vi "Init PAS CVT.vi"(8 "error in":errorcluster, 10 "CVT Session in":T2, 11 "Cfg Ref in":T1) -> (0 "error out":errorcluster, 2 "CVT Session Out":T2, 3 "Refnum out":T1)   [LabVIEW 2014, in "Controller.lvlib" / "Controller.lvclass"]
uses:
  Controller.lvclass
  <userlib>/_Session Fwk/Typedefs/Session Handle.ctl
  <userlib>/_Session Fwk/Session - Root.lvclass
  <vilib>/Utility/config.llb/Config Data RefNum.ctl
  <vilib>/Utility/config.llb/Read Key (Boolean).vi
  <vilib>/Utility/config.llb/Read Key (I32).vi
  <vilib>/Utility/config.llb/Read Key (Double).vi
  <vilib>/Utility/config.llb/Read Key (String).vi
  <vilib>/Utility/config.llb/NI_LVConfig.lvlib
  reusable/Session APIs/CVT/CVT.lvclass
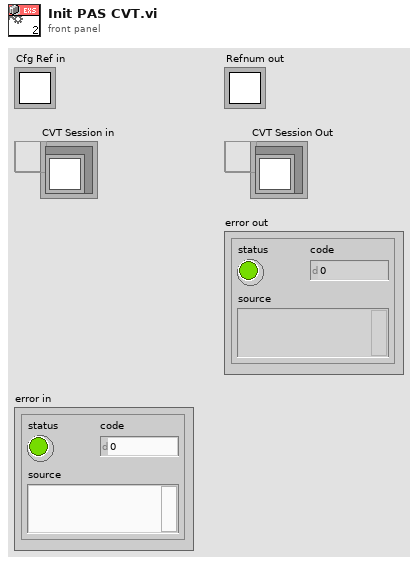
[diagram p1: front panel]
types:
  T1 = typedef "NI_LVConfig.lvlib/Config Data RefNum.ctl" = refnum<k1>
  T2 = typedef "Session - Root.lvclass/Session Handle.ctl" = refnum<data-value>
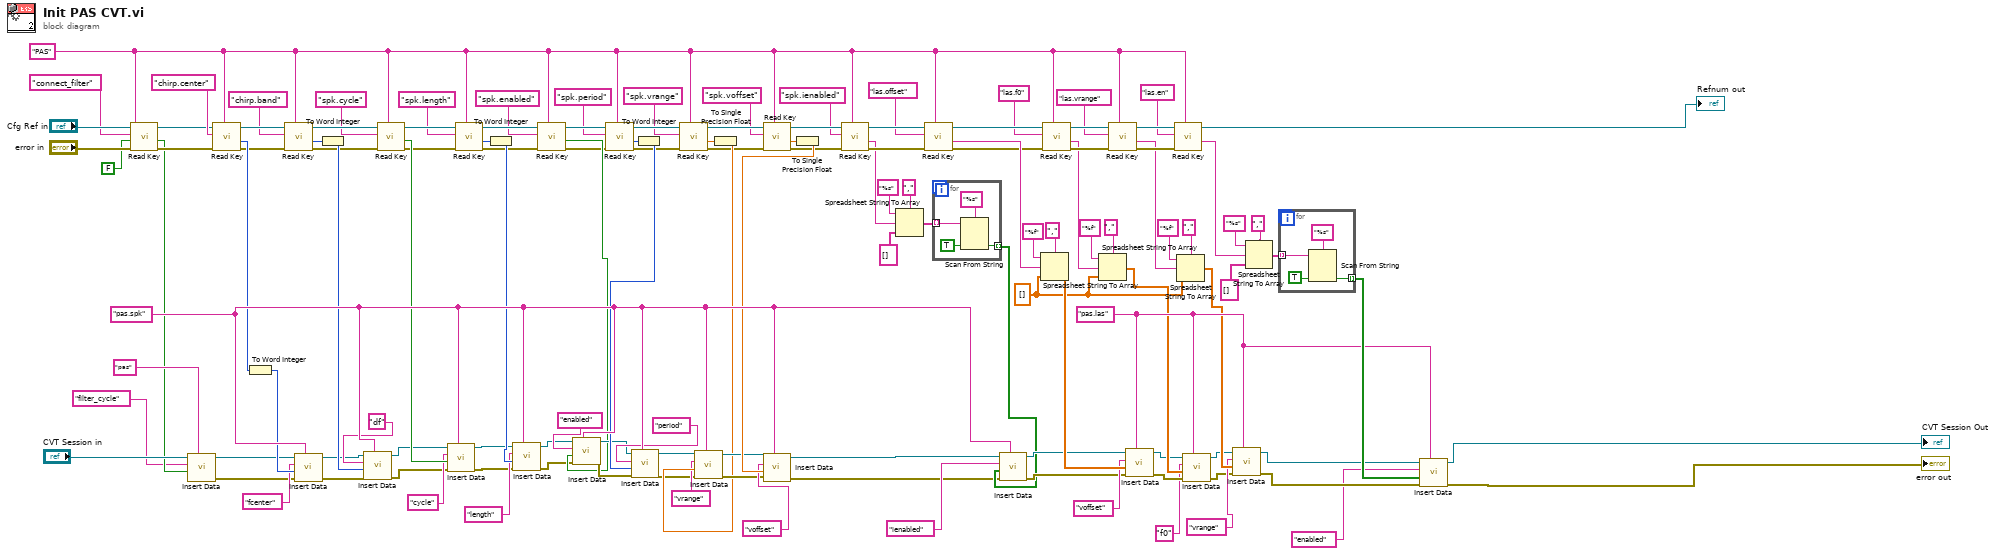
[diagram p0: block diagram]
diagram:
  w13 = "PAS" ("section")
  w125 = "pas.las" ("Group")
  w108 = "pas.spk" ("Group")
  w76 = sgl[] []
  n1 = call-poly <vilib>:"Read Key.vi"("section"=w13, "error in (no error)"="error in", "default value"=FALSE, "key"="connect_filter", "refnum"="Cfg Ref in") -> ("error out"=w9:errorcluster, "value"=w4:bool, "refnum out"=w10:T1)  [unwired: 3 in, 1 out]
  n2 = call "Insert Data.vi"("Group"="pas", "Data"=w4, "tag"="filter_cycle", "CVT Session In"="CVT Session in") -> ("error out"=w1:errorcluster, "CVT Session Out"=w2:T2)  [unwired: 6 in]
  n3 = call-poly <vilib>:"Read Key.vi"("section"=w13, "error in (no error)"=w9, "key"="chirp.center", "refnum"=w10) -> ("error out"=w54:errorcluster, "value"=w57:i32, "refnum out"=w56:T1)  [unwired: 4 in, 1 out]
  n4 = To Word Integer(number=w57) -> (16bit integer=w78:i16)
  n5 = call-poly <vilib>:"Read Key.vi"("section"=w13, "error in (no error)"=w54, "key"="chirp.band", "refnum"=w56) -> ("error out"=w51:errorcluster, "value"=w53:i32, "refnum out"=w52:T1)  [unwired: 4 in, 1 out]
  n6 = call "Insert Data.vi"("Group"=w108, "error in"=w1, "Data"=w78, "tag"="fcenter", "CVT Session In"=w2) -> ("error out"=w131:errorcluster, "CVT Session Out"=w79:T2)  [unwired: 5 in]
  n7 = To Word Integer(number=w53) -> (16bit integer=w80:i16)
  n8 = call "Insert Data.vi"("Group"=w108, "error in"=w131, "Data"=w80, "tag"="df", "CVT Session In"=w79) -> ("error out"=w83:errorcluster, "CVT Session Out"=w82:T2)  [unwired: 5 in]
  n9 = call-poly <vilib>:"Read Key.vi"("section"=w13, "error in (no error)"=w51, "key"="spk.cycle", "refnum"=w52) -> ("error out"=w60:errorcluster, "value"=w85:bool, "refnum out"=w59:T1)  [unwired: 4 in, 1 out]
  n10 = call "Insert Data.vi"("Group"=w108, "error in"=w83, "Data"=w85, "tag"="cycle", "CVT Session In"=w82) -> ("error out"=w87:errorcluster, "CVT Session Out"=w86:T2)  [unwired: 5 in]
  n11 = call-poly <vilib>:"Read Key.vi"("section"=w13, "error in (no error)"=w60, "key"="spk.length", "refnum"=w59) -> ("error out"=w45:errorcluster, "value"=w47:i32, "refnum out"=w61:T1)  [unwired: 4 in, 1 out]
  n12 = To Word Integer(number=w47) -> (16bit integer=w89:i16)
  n13 = call "Insert Data.vi"("Group"=w108, "error in"=w87, "Data"=w89, "tag"="length", "CVT Session In"=w86) -> ("error out"=w91:errorcluster, "CVT Session Out"=w90:T2)  [unwired: 5 in]
  n14 = call-poly <vilib>:"Read Key.vi"("section"=w13, "error in (no error)"=w45, "key"="spk.enabled", "refnum"=w61) -> ("error out"=w62:errorcluster, "value"=w93:bool, "refnum out"=w65:T1)  [unwired: 4 in, 1 out]
  n15 = call "Insert Data.vi"("Group"=w108, "error in"=w91, "Data"=w93, "tag"="enabled", "CVT Session In"=w90) -> ("error out"=w97:errorcluster, "CVT Session Out"=w94:T2)  [unwired: 5 in]
  n16 = call-poly <vilib>:"Read Key.vi"("section"=w13, "error in (no error)"=w62, "key"="spk.period", "refnum"=w65) -> ("error out"=w63:errorcluster, "value"=w46:i32, "refnum out"=w66:T1)  [unwired: 4 in, 1 out]
  n17 = To Word Integer(number=w46) -> (16bit integer=w96:i16)
  n18 = call "Insert Data.vi"("Group"=w108, "error in"=w97, "Data"=w96, "tag"="period", "CVT Session In"=w94) -> ("error out"=w99:errorcluster, "CVT Session Out"=w98:T2)  [unwired: 5 in]
  n19 = call-poly <vilib>:"Read Key.vi"("section"=w13, "error in (no error)"=w63, "key"="spk.vrange", "refnum"=w66) -> ("error out"=w42:errorcluster, "value"=w40:dbl, "refnum out"=w43:T1)  [unwired: 4 in, 1 out]
  n20 = To Single Precision Float(number=w40) -> (single precision float=w101:sgl)
  n21 = call "Insert Data.vi"("Group"=w108, "error in"=w99, "Data"=w101, "tag"="vrange", "CVT Session In"=w98) -> ("error out"=w102:errorcluster, "CVT Session Out"=w103:T2)  [unwired: 5 in]
  n22 = call-poly <vilib>:"Read Key.vi"("section"=w13, "error in (no error)"=w42, "key"="spk.voffset", "refnum"=w43) -> ("error out"=w73:errorcluster, "value"=w41:dbl, "refnum out"=w72:T1)  [unwired: 4 in, 1 out]
  n23 = To Single Precision Float(number=w41) -> (single precision float=w105:sgl)
  n24 = call "Insert Data.vi"("Group"=w108, "error in"=w102, "Data"=w105, "tag"="voffset" ("key"), "CVT Session In"=w103) -> ("error out"=w107:errorcluster, "CVT Session Out"=w106:T2)  [unwired: 5 in]
  n25 = call-poly <vilib>:"Read Key.vi"("section"=w13, "error in (no error)"=w73, "key"="spk.ienabled", "refnum"=w72) -> ("error out"=w68:errorcluster, "value"=w14:string, "refnum out"=w67:T1)  [unwired: 4 in, 1 out]
  n26 = Spreadsheet String To Array(delimiter (Tab)=",", format string="%s", spreadsheet string=w14, array type (2D Dbl)=string[] []) -> (array=w18:string[])
  n27 = call-poly <vilib>:"Read Key.vi"("section"=w13, "error in (no error)"=w68, "key"="las.offset", "refnum"=w67) -> ("error out"=w29:errorcluster, "value"=w64:string, "refnum out"=w30:T1)  [unwired: 4 in, 1 out]
  n28 = for {
    tunnel: w18 -> [w135] mode=indexing
    tunnel: [w132] -> w110 mode=indexing
    n29 = Scan From String(format string="%s", input string=w135, default 1=TRUE) -> (output 1=w132:bool)  [unwired: 2 in, 3 out]
  }
  n30 = call "Insert Data.vi"("Group"=w108, "error in"=w107, "Data"=w110, "tag"="ienabled" ("key"), "CVT Session In"=w106) -> ("error out"=w112:errorcluster, "CVT Session Out"=w111:T2)  [unwired: 5 in]
  n31 = Spreadsheet String To Array(delimiter (Tab)=",", format string="%f", spreadsheet string=w64, array type (2D Dbl)=w76) -> (array=w114:sgl[])
  n32 = call-poly <vilib>:"Read Key.vi"("section"=w13, "error in (no error)"=w29, "key"="las.f0", "refnum"=w30) -> ("error out"=w75:errorcluster, "value"=w69:string, "refnum out"=w74:T1)  [unwired: 4 in, 1 out]
  n33 = Spreadsheet String To Array(delimiter (Tab)=",", format string="%f", spreadsheet string=w69, array type (2D Dbl)=w76) -> (array=w118:sgl[])
  n34 = call-poly <vilib>:"Read Key.vi"("section"=w13, "error in (no error)"=w75, "key"="las.vrange", "refnum"=w74) -> ("error out"=w71:errorcluster, "value"=w36:string, "refnum out"=w70:T1)  [unwired: 4 in, 1 out]
  n35 = call "Insert Data.vi"("Group"=w125, "error in"=w112, "Data"=w114, "tag"="voffset" ("Tag Name"), "CVT Session In"=w111) -> ("error out"=w117:errorcluster, "CVT Session Out"=w116:T2)  [unwired: 5 in]
  n36 = call-poly <vilib>:"Read Key.vi"("section"=w13, "error in (no error)"=w71, "key"="las.en", "refnum"=w70) -> ("value"=w21:string, "refnum out"=→"Refnum out":T1)  [unwired: 4 in, 2 out]
  n37 = Spreadsheet String To Array(delimiter (Tab)=",", format string="%f", spreadsheet string=w36, array type (2D Dbl)=w76) -> (array=w122:sgl[])
  n38 = call "Insert Data.vi"("Group"=w125, "error in"=w117, "Data"=w118, "tag"="f0", "CVT Session In"=w116) -> ("error out"=w120:errorcluster, "CVT Session Out"=w119:T2)  [unwired: 5 in]
  n39 = call "Insert Data.vi"("Group"=w125, "error in"=w120, "Data"=w122, "tag"="vrange" ("key"), "CVT Session In"=w119) -> ("error out"=w127:errorcluster, "CVT Session Out"=w123:T2)  [unwired: 5 in]
  n40 = Spreadsheet String To Array(delimiter (Tab)=",", format string="%s", spreadsheet string=w21, array type (2D Dbl)=string[] []) -> (array=w22:string[])
  n41 = for {
    tunnel: w22 -> [w139] mode=indexing
    tunnel: [w136] -> w126 mode=indexing
    n42 = Scan From String(format string="%s", input string=w139, default 1=TRUE) -> (output 1=w136:bool)  [unwired: 2 in, 3 out]
  }
  n43 = call "Insert Data.vi"("Group"=w125, "error in"=w127, "Data"=w126, "tag"="enabled" ("Tag Name"), "CVT Session In"=w123) -> ("error out"=→"error out":errorcluster, "CVT Session Out"=→"CVT Session Out":T2)  [unwired: 5 in]
